vi "MoveAnalyserNotInUse.vi"(6 "Analysers Motor Control":T2=enum."Get Angle", 9 "file (use dialog)":path, 11 "Analyser Set Angles":cluster{"Analyser 1":i32, "Analyser 2":i32}) -> (0 "Found Home?":cluster{"Analyser 1":bool, "Analyser 2":bool}, 1 "Analysers Moving?":T1, 2 "Crenelation \nInterrupts":bool[](array[boolean]) caption="Crenelation Indicators", 3 "Current Angles":cluster{"Analyser 1":i32, "Analyser 2":i32})   [LabVIEW 2014]
uses:
  typedef_analyser_motor_control.ctl
  Timer/typedef_timer.ctl
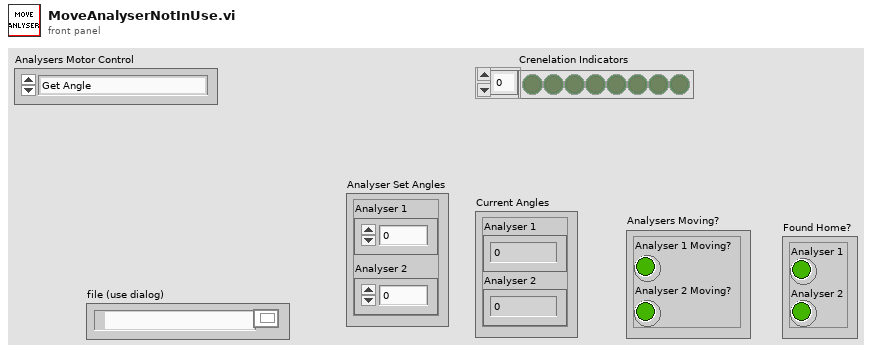
[diagram p1: front panel]
types:
  T1 = cluster{"Analyser 1 Moving?":bool, "Analyser 2 Moving?":bool}
  T2 = typedef "typedef_analyser_motor_control.ctl" = enum16{"Run", "A1 Find 45 Deg Postively", "A1 Find 45 Deg Negatively", "A2 Find 45 Deg Positively", "A2 Find 45 Deg Negatively", "Get Angle", "Set Angle"}
  T3 = typedef "typedef_timer.ctl" = enum16{"Reset", "Initialise", "Timed Out & Reset", "Timed Out"}
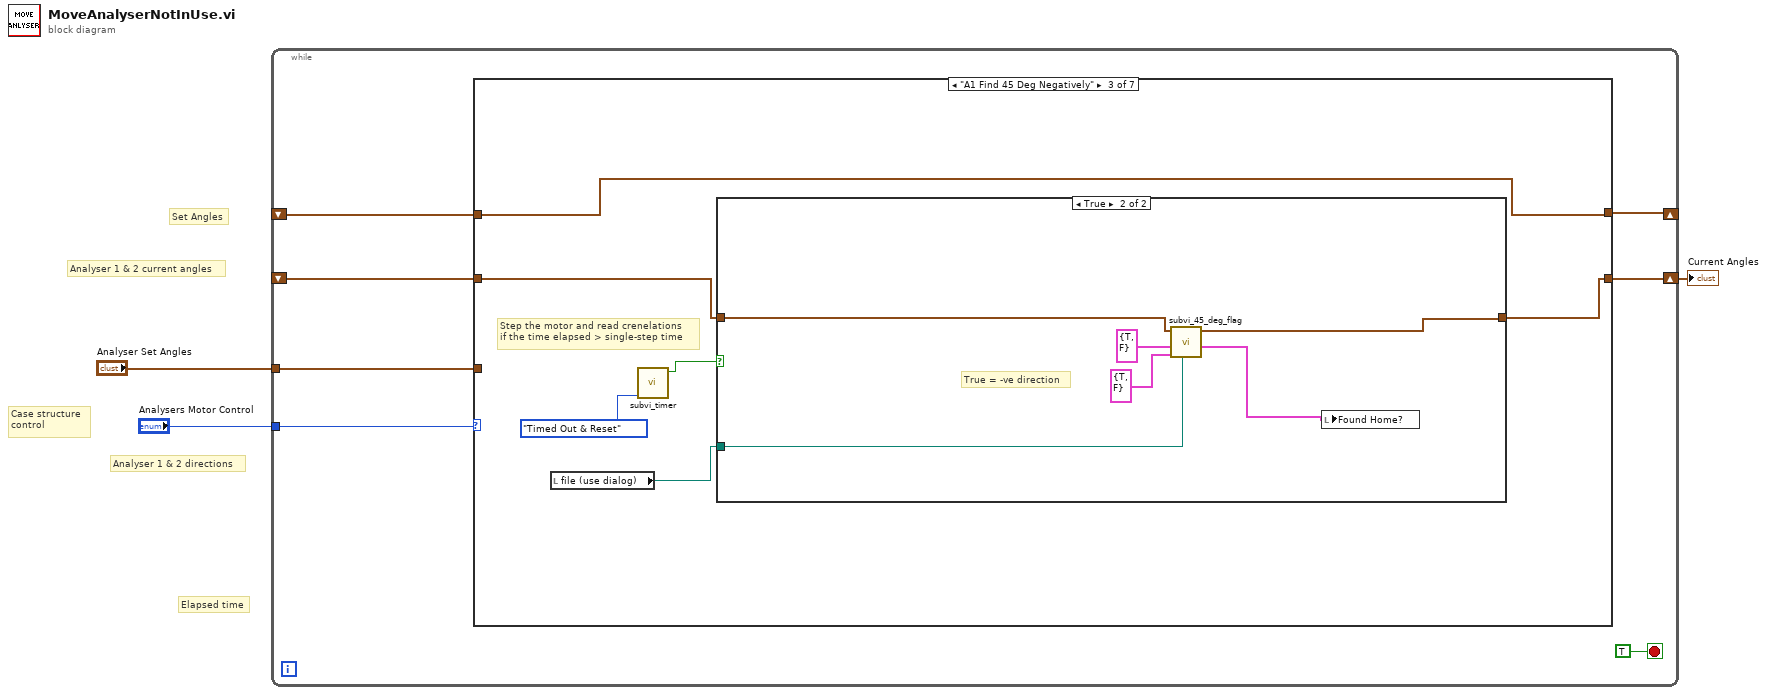
[diagram p0: block diagram]
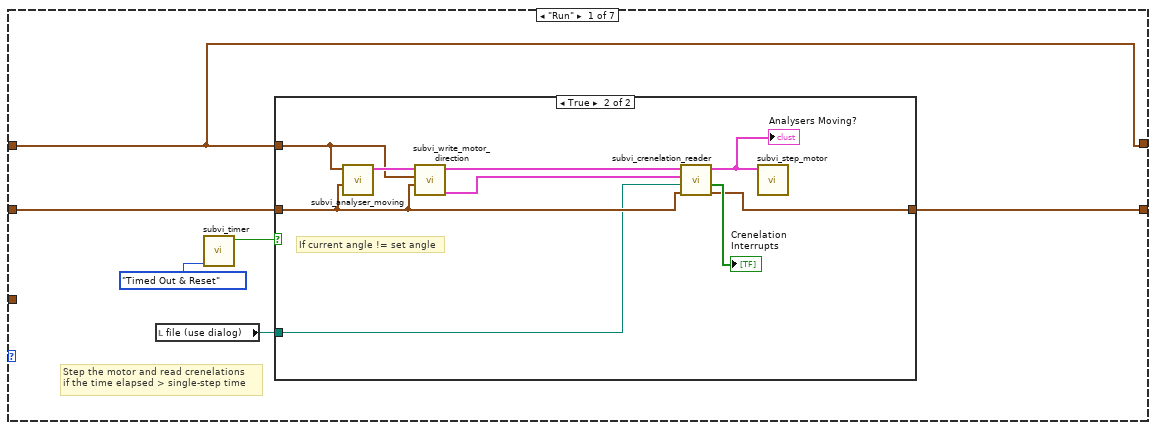
[diagram p2: hidden frame]
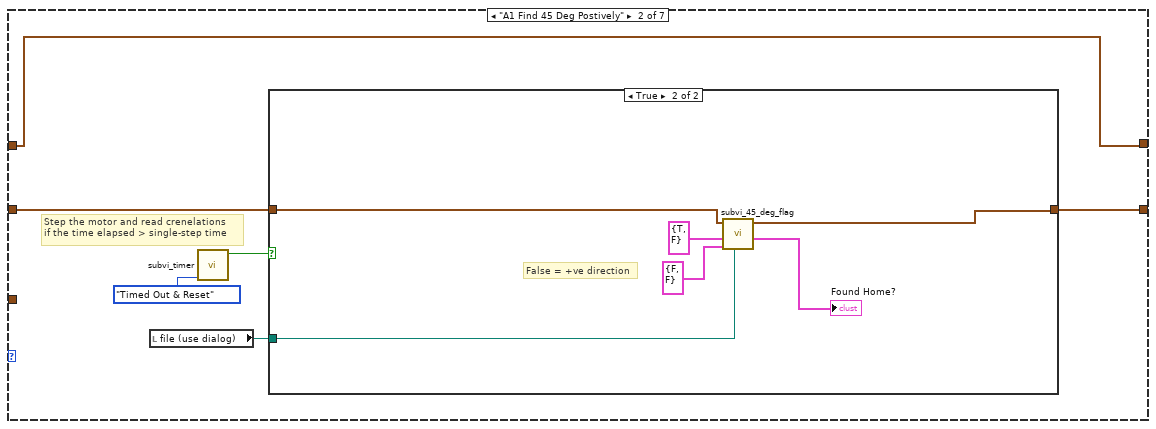
[diagram p4: hidden frame]
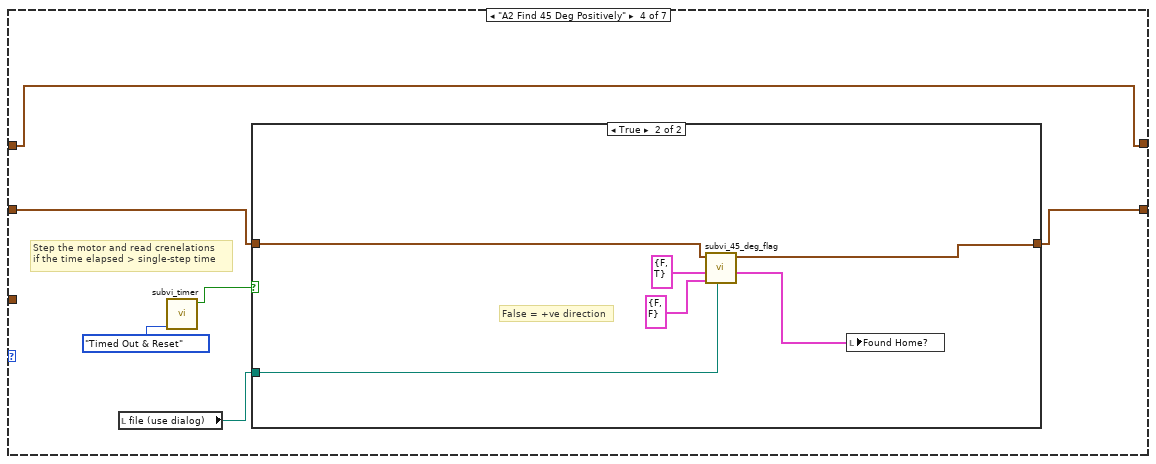
[diagram p7: hidden frame]
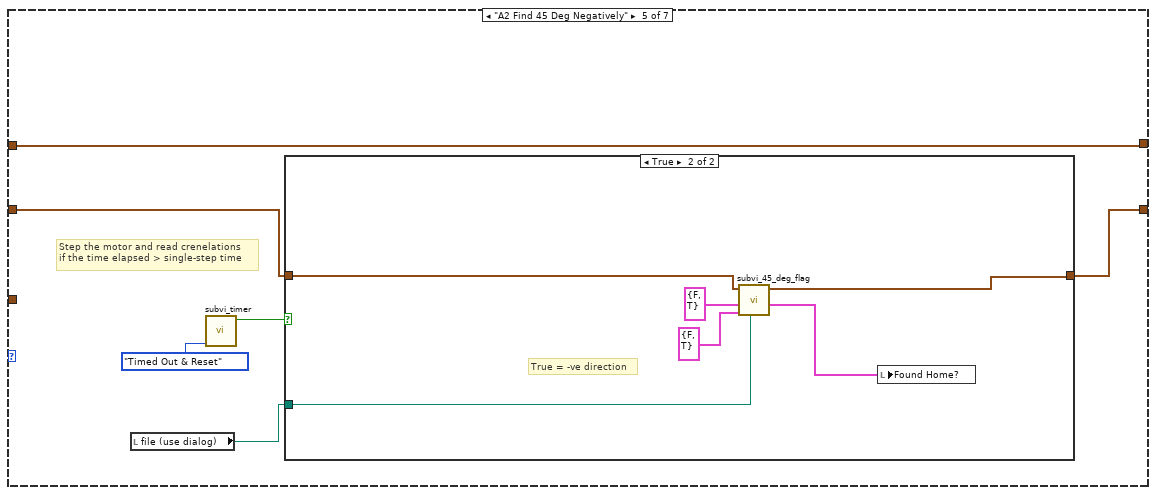
[diagram p9: hidden frame]
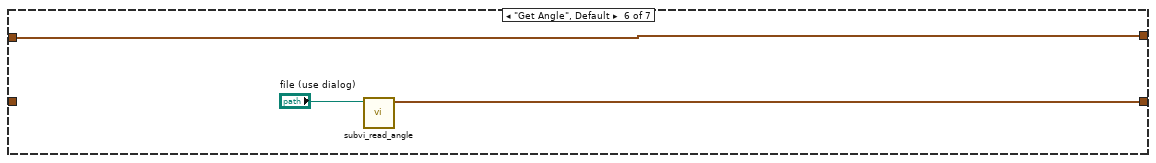
[diagram p11: hidden frame]
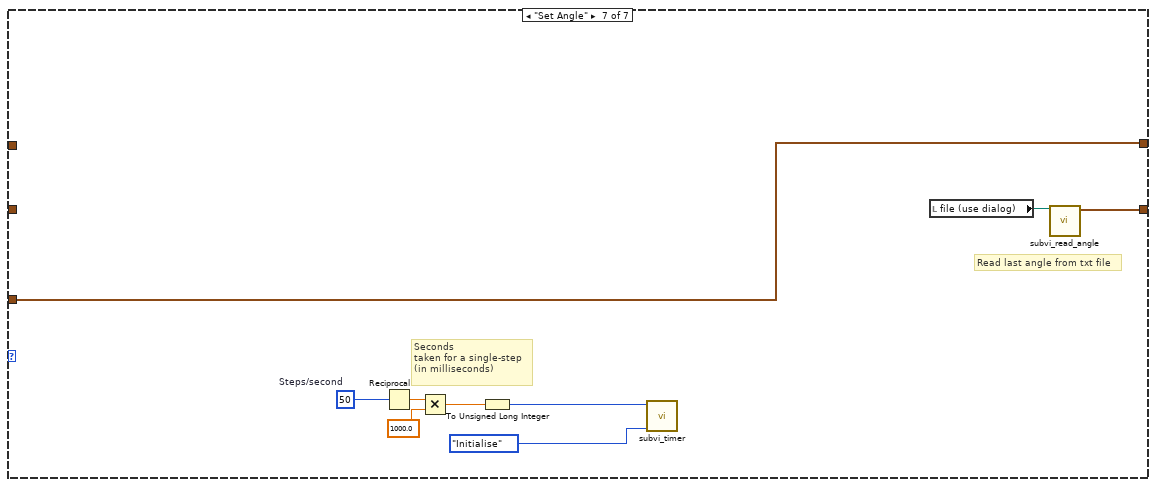
[diagram p12: hidden frame]
diagram:
  # "Set Angles"
  # "Analyser 1 & 2 directions"
  # "Elapsed time"
  # "Analyser 1 & 2 current angles"
  # "Case structure \ncontrol"
  n1 = while {
    tunnel: "Analysers Motor Control" -> [w10]
    shift-right: [w9] -> w1
    shift-left: _ -> [w8]
    shift-right: [w5] -> _
    shift-left: _ -> [w7]
    tunnel: "Analyser Set Angles" -> [w4]
    stop <- TRUE stop-if-true
    n2 = case shown="\"A1 Find 45 Deg Negatively\"" w10 {
      tunnel: [w11 w27 w41 w54 w66 w80 w83] -> w9
      tunnel: w8 -> [w12 w28 w42 w57 w70 _ _]
      tunnel: w7 -> [w13 w29 w40 w53 w67 w79 _]
      tunnel: [w13 w29 w40 w53 w67 w79 w90] -> w5
      tunnel: w4 -> [_ _ _ _ _ _ w90]
      frame "Run" {
        # "Step the motor and read crenelations \nif the time elapsed > single-step time"
        n3 = local read "file (use dialog)"() -> (w14:path)
        n4 = call "subvi_timer.vi"("Timer Functions"=typedef_timer."Timed Out & Reset") -> ("Timed Out?"=w15:bool)  [unwired: 9 in, 1 out]
        n5 = case shown="True" w15 {
          tunnel: w12 -> [w17 w24]
          tunnel: w13 -> [_ w25]
          tunnel: w14 -> [_ w21]
          tunnel: [w17 w18] -> w11
          frame False {
          }
          frame True {
            # "If current angle != set angle"
            n6 = call "subvi_analyser_moving.vi"("Current Angles"=w24, "Set Angles"=w25) -> ("Analysers Moving?"=w26:T1)  [unwired: 9 in]
            n7 = call "subvi_write_motor_direction.vi"("Current Angles"=w24, "Set Angles"=w25, "Analysers Moving?"=w26) -> ("Directions"=w22:cluster{"Analyser 1":bool, "Analyser 2":bool}, "Analysers Moving? Output"=w23:T1)  [unwired: 7 in]
            n8 = call "subvi_crenelation_reader.vi"("Current Angles"=w24, "file (use dialog) 2"=w21, "Directions"=w22, "Analysers Moving?"=w23) -> ("New Current Angles"=w18:cluster{"Analyser 1":i32, "Analyser 2":i32}, "Crenelation \nInterrupts"=→"Crenelation \nInterrupts":bool[], "Analysers Moving? Output"=w20:T1)  [unwired: 5 in]
            "Analysers Moving?" <- w20
            n9 = call "subvi_step_motor.vi"("Write to Motor?"=w20) -> ()  [unwired: 11 in]
          }
        }
      }
      frame "A1 Find 45 Deg Postively" {
        # "Step the motor and read crenelations \nif the time elapsed > single-step time"
        n10 = local read "file (use dialog)"() -> (w30:path)
        n11 = call "subvi_timer.vi"("Timer Functions"=typedef_timer."Timed Out & Reset") -> ("Timed Out?"=w31:bool)  [unwired: 9 in, 1 out]
        n12 = case shown="True" w31 {
          tunnel: w30 -> [_ w36]
          tunnel: w28 -> [w33 w37]
          tunnel: [w33 w35] -> w27
          frame False {
          }
          frame True {
            # "False = +ve direction"
            n13 = call "subvi_45_deg_flag.vi"("file (use dialog)"=w36, "Directions"=cluster{"Analyser 1":bool, "Analyser 2":bool} {"Analyser 1"=FALSE, "Analyser 2"=FALSE}, "Analysers Moving?"=T1 {"Analyser 1 Moving?"=TRUE, "Analyser 2 Moving?"=FALSE}, "Current Angles"=w37) -> ("Found Home?"=→"Found Home?":cluster{"Analyser 1":bool, "Analyser 2":bool}, "New Current Angles"=w35:cluster{"Numeric Control":i32, "Analyser 2":i32})  [unwired: 6 in]
          }
        }
      }
      frame "A1 Find 45 Deg Negatively" {
        # "Step the motor and read crenelations \nif the time elapsed > single-step time"
        n14 = local read "file (use dialog)"() -> (w43:path)
        n15 = call "subvi_timer.vi"("Timer Functions"=typedef_timer."Timed Out & Reset") -> ("Timed Out?"=w45:bool)  [unwired: 9 in, 1 out]
        n16 = case shown="True" w45 {
          tunnel: w43 -> [_ w49]
          tunnel: w42 -> [w46 w50]
          tunnel: [w46 w48] -> w41
          frame False {
          }
          frame True {
            # "True = -ve direction"
            n17 = call "subvi_45_deg_flag.vi"("file (use dialog)"=w49, "Directions"=cluster{"Analyser 1":bool, "Analyser 2":bool} {"Analyser 1"=TRUE, "Analyser 2"=FALSE}, "Analysers Moving?"=T1 {"Analyser 1 Moving?"=TRUE, "Analyser 2 Moving?"=FALSE}, "Current Angles"=w50) -> ("Found Home?"=w47:cluster{"Analyser 1":bool, "Analyser 2":bool}, "New Current Angles"=w48:cluster{"Numeric Control":i32, "Analyser 2":i32})  [unwired: 6 in]
            n18 = local write "Found Home?"(w47) -> ()
          }
        }
      }
      frame "A2 Find 45 Deg Positively" {
        # "Step the motor and read crenelations \nif the time elapsed > single-step time"
        n19 = local read "file (use dialog)"() -> (w55:path)
        n20 = call "subvi_timer.vi"("Timer Functions"=typedef_timer."Timed Out & Reset") -> ("Timed Out?"=w56:bool)  [unwired: 9 in, 1 out]
        n21 = case shown="True" w56 {
          tunnel: w55 -> [_ w62]
          tunnel: w57 -> [w59 w63]
          tunnel: [w59 w61] -> w54
          frame False {
          }
          frame True {
            # "False = +ve direction"
            n22 = call "subvi_45_deg_flag.vi"("file (use dialog)"=w62, "Directions"=cluster{"Analyser 1":bool, "Analyser 2":bool} {"Analyser 1"=FALSE, "Analyser 2"=FALSE}, "Analysers Moving?"=T1 {"Analyser 1 Moving?"=FALSE, "Analyser 2 Moving?"=TRUE}, "Current Angles"=w63) -> ("Found Home?"=w60:cluster{"Analyser 1":bool, "Analyser 2":bool}, "New Current Angles"=w61:cluster{"Numeric Control":i32, "Analyser 2":i32})  [unwired: 6 in]
            n23 = local write "Found Home?"(w60) -> ()
          }
        }
      }
      frame "A2 Find 45 Deg Negatively" {
        # "Step the motor and read crenelations \nif the time elapsed > single-step time"
        n24 = local read "file (use dialog)"() -> (w68:path)
        n25 = call "subvi_timer.vi"("Timer Functions"=typedef_timer."Timed Out & Reset") -> ("Timed Out?"=w69:bool)  [unwired: 9 in, 1 out]
        n26 = case shown="True" w69 {
          tunnel: w68 -> [_ w75]
          tunnel: w70 -> [w72 w76]
          tunnel: [w72 w74] -> w66
          frame False {
          }
          frame True {
            # "True = -ve direction"
            n27 = call "subvi_45_deg_flag.vi"("file (use dialog)"=w75, "Directions"=cluster{"Analyser 1":bool, "Analyser 2":bool} {"Analyser 1"=FALSE, "Analyser 2"=TRUE}, "Analysers Moving?"=T1 {"Analyser 1 Moving?"=FALSE, "Analyser 2 Moving?"=TRUE}, "Current Angles"=w76) -> ("Found Home?"=w73:cluster{"Analyser 1":bool, "Analyser 2":bool}, "New Current Angles"=w74:cluster{"Numeric Control":i32, "Analyser 2":i32})  [unwired: 6 in]
            n28 = local write "Found Home?"(w73) -> ()
          }
        }
      }
      frame "Get Angle", Default {
        n29 = call "subvi_read_angle.vi"("file (use dialog)"="file (use dialog)") -> ("Current Angles"=w80:cluster{"Analyser 1":i32, "Analyser 2":i32})  [unwired: 10 in]
      }
      frame "Set Angle" {
        w88 = 50  # Steps/second
        # "Read last angle from txt file"
        # "Seconds \ntaken for a single-step\n(in milliseconds)"
        n30 = Reciprocal(x=w88) -> (1/x=w87:dbl)
        n31 = Multiply(x=w87, y=1000.0) -> (x*y=w85:dbl)
        n32 = To Unsigned Long Integer(number=w85) -> (unsigned 32bit integer=w84:u32)
        n33 = call "subvi_timer.vi"("Timer Functions"=typedef_timer."Initialise", "Threshold Time (ms)"=w84) -> ()  [unwired: 8 in, 2 out]
        n34 = local read "file (use dialog)"() -> (w82:path)
        n35 = call "subvi_read_angle.vi"("file (use dialog)"=w82) -> ("Current Angles"=w83:cluster{"Analyser 1":i32, "Analyser 2":i32})  [unwired: 10 in]
      }
    }
  }
  "Current Angles" <- w1
